vi "CheesyDrive.vi"(6 "Quickturn":bool, 7 "SlowMode":u32, 8 "Fast Mode":bool, 10 "Wheel":dbl(slide)=-0.015748031496062992 scale=-1.0..1.0, 11 "Throttle":dbl(slide)=0.007874015748031496 scale=-1.0..1.0) -> (2 "Right PWM":dbl, 3 "Left PWM":dbl)   [LabVIEW 2018]
doc: "Implements CheesyDrive. CheesyDrive means that the turn joystick controls the radius of turning instead of the rate of turning. Also implements QuickStop and QuickTurn."
uses:
  Robot-Project/Arm/Implementation/Arm Published Globals.vi
panel:
  in  "ArrayOfSlownesss":T1(array[cluster])=[{"MaxSpeedSlow"=1.0, "SlowRate"=5.0, "MaxTurnSlow"=1.0, "MaxTurnRateSlow"=8.0}, {"MaxSpeedSlow"=0.6, "SlowRate"=4.0, "MaxTurnSlow"=0.8, "MaxTurnRateSlow"=10.0}, {"MaxSpeedSlow"=0.4, "SlowRate"=3.0, "MaxTurnSlow"=0.75, "MaxTurnRateSlow"=10.0}]
  in  "PointsTurn":cluster{"X":dbl, "Y":dbl}[](array[cluster])=[{"X"=0.0, "Y"=0.0}, {"X"=0.04, "Y"=0.0}, {"X"=0.041, "Y"=0.01}, {"X"=0.6, "Y"=0.3}, {"X"=1.0, "Y"=1.0}]
  in  "PointsQuickTurn":cluster{"X":dbl, "Y":dbl}[](array[cluster])=[{"X"=0.0, "Y"=0.0}, {"X"=0.05, "Y"=0.05}, {"X"=1.0, "Y"=0.6}]
  in  "PointsThrottle":cluster{"X":dbl, "Y":dbl}[](array[cluster])=[{"X"=0.0, "Y"=0.0}, {"X"=0.025, "Y"=0.0}, {"X"=1.0, "Y"=0.75}]
  in  "QSMult":dbl=0.12
  in  "WheelNonLinearity":dbl=0.01
  in  "negInertiaScalar":dbl=4.0
  in  "alpha":dbl=0.1
  out "QuickStop Value":dbl(graph)
  in  "Sensitivty":dbl=1.0
  # "These are the inputs and outputs\nNot configuration"
  # "Check block diagram for details on these"
  # "normal"
  # "Switch"
  # "Scale"
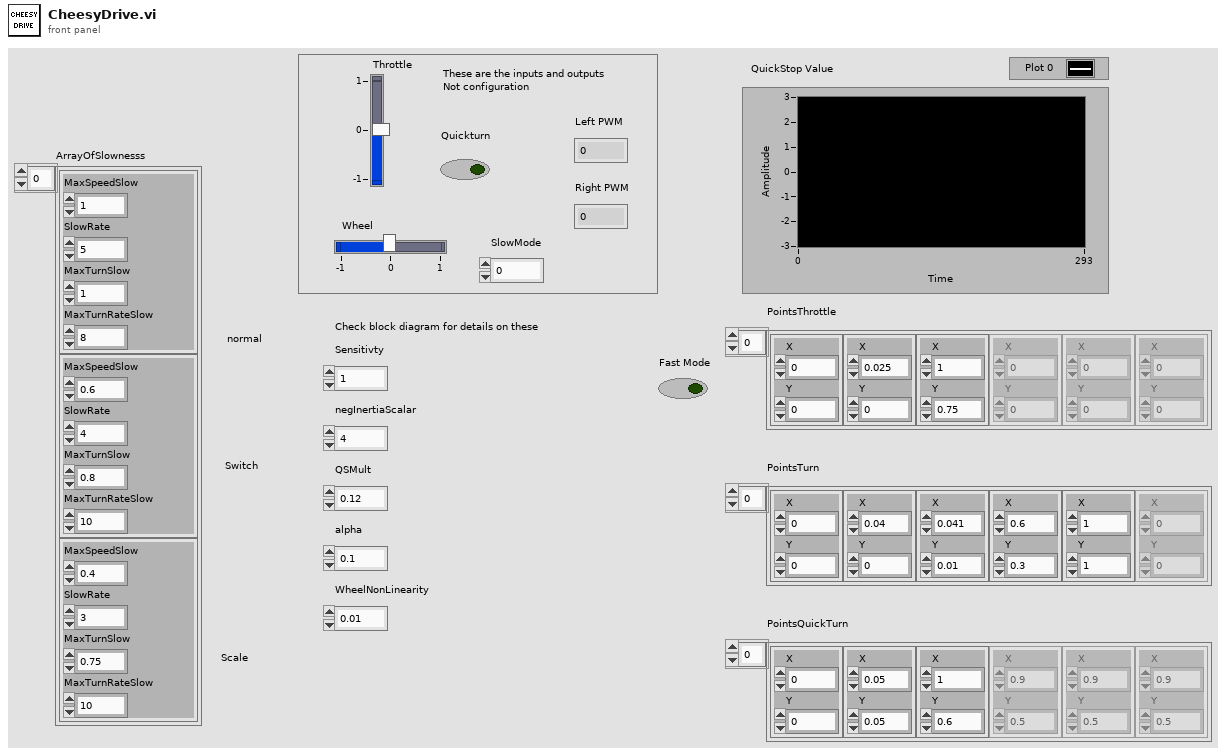
[diagram p1: front panel]
types:
  T1 = cluster{"MaxSpeedSlow":dbl, "SlowRate":dbl, "MaxTurnSlow":dbl, "MaxTurnRateSlow":dbl}[]
  T2 = cluster{"MaxSpeedSlow":dbl, "SlowRate":dbl, "MaxTurnSlow":dbl, "MaxTurnRateSlow":dbl}
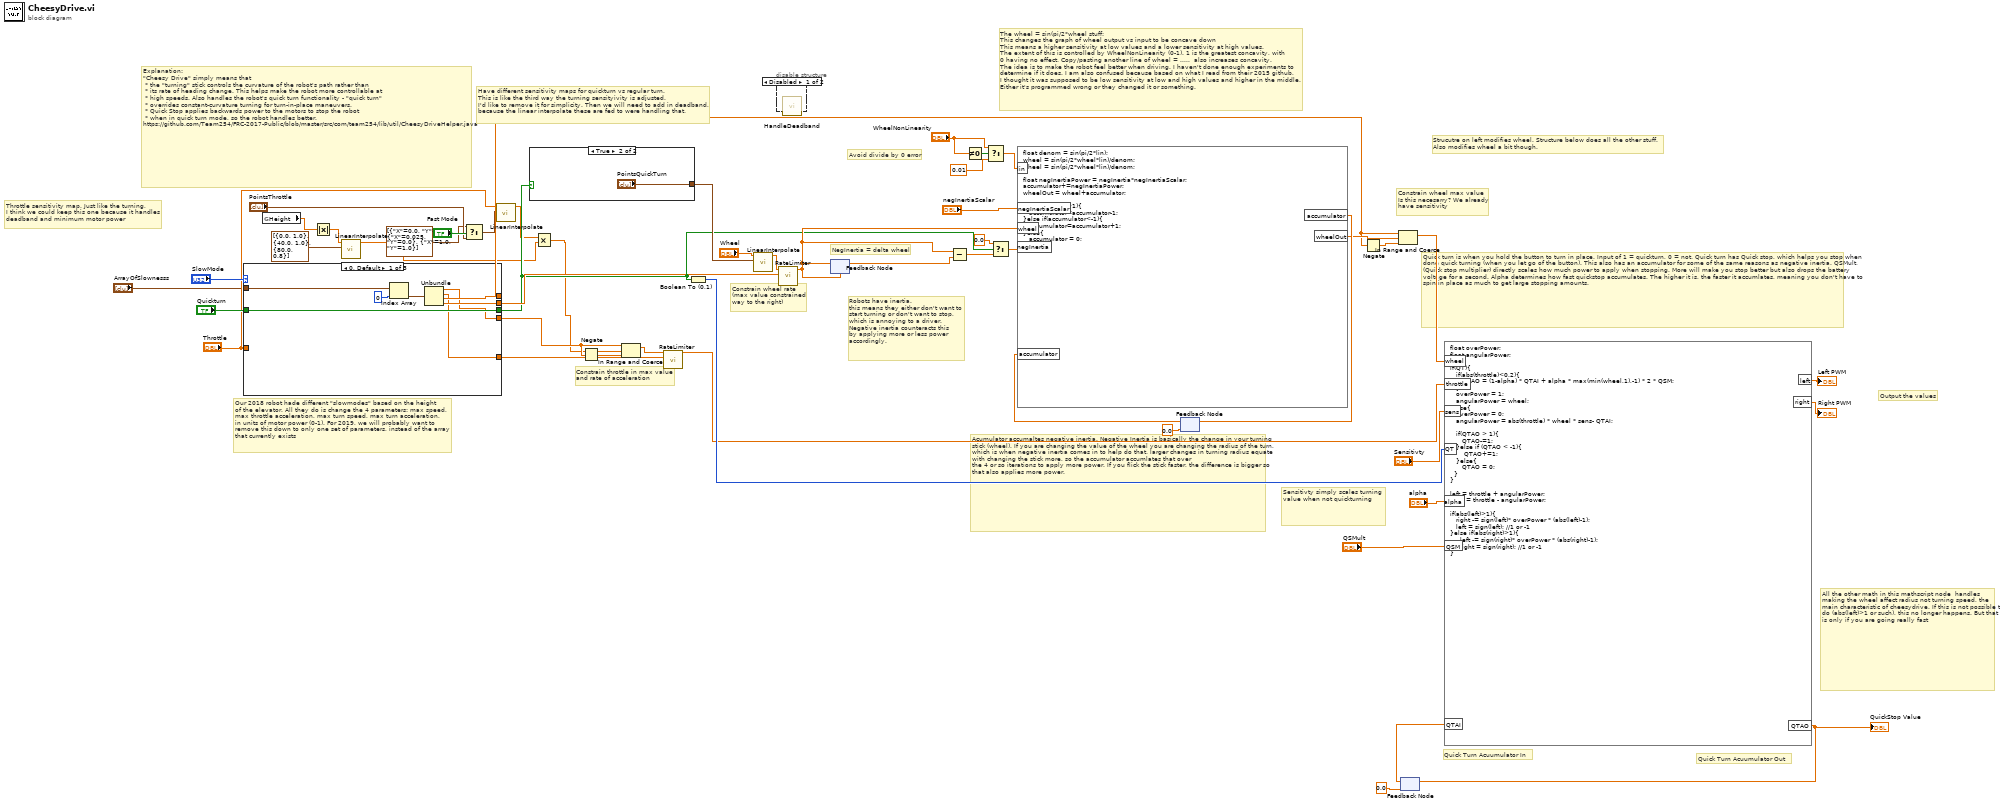
[diagram p0: block diagram]
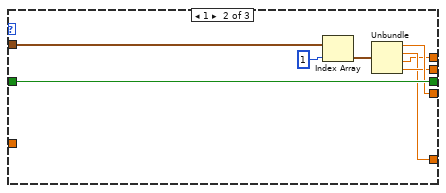
[diagram p3: hidden frame]
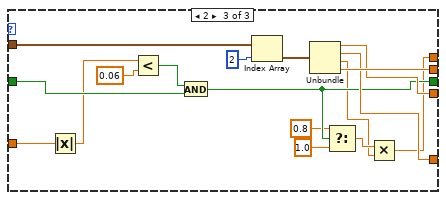
[diagram p4: hidden frame]
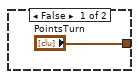
[diagram p5: hidden frame]
diagram:
  # "Strucutre on left modifies wheel. Structure below does all the other stuff.\nAlso modifies wheel a bit though."
  # "Sensitivty simply scales turning value when not quickturning"
  # "All the other math in this mathscript node  handles making the wheel affect radius not turning speed, the main characteristic of cheesydrive. If this is not possible to do (abs(left)>1 or such), this no longer happens. But that is only if you are going really fast"
  # "Quick turn is when you hold the button to turn in place. Input of 1 = quickturn, 0 = not. Quick turn has Quick stop, which helps you stop when done quick turning (when you let go of the button). This also has an accumulator for some of the same reasons as negative inertia. QSMult, (Quick stop multiplier) directly scales how much power to apply when stopping. More will make you stop better but also drops the battery voltage for a second. Alpha determines how fast quickstop accumulates. The higher it is, the faster it accumlates, meaning you don't have to spin in place as much to get large stopping amounts."
  # "Output the values"
  # "Acumulator accumaltes negative inertia. Negative Inertia is basically the change in your turning stick (wheel). If you are changing the value of the wheel you are changing the radius of the turn, which is when negative inertia comes in to help do that. larger changes in turning radius equate with changing the stick more, so the accumulator accumlates that over\nthe 4 or so iterations to apply more power. If you flick the stick faster, the difference is bigger so that also applies more power."
  # "The wheel = sin(pi/2*wheel stuff:\nThis changes the graph of wheel output vs input to be concave down\nThis means a higher sensitivity at low values and a lower sensitivity at high values.\nThe extent of this is controlled by WheelNonLinearity (0-1). 1 is the greatest concavity, with\n0 having no effect. Copy/pasting another line of wheel = .....  also increases concavity.\nThe idea is to make the robot feel better when driving. I haven't done enough experiments to \ndetermine if it does. I am also confused because based on what I read from their 2015 github,\nI thought it was supposed to be low sensitivity at low and high values and higher in the middle.\nEither it's programmed wrong or they changed it or something."
  # "Constrain wheel max value\nIs this necesarry? We already\nhave sensitivity"
  # "Constrain wheel rate\n(max value constrained\nway to the right)"
  # "Throttle sensitivity map. Just like the turning,\nI think we could keep this one because it handles\ndeadband and minimum motor power"
  # "Have different sensitivity maps for quickturn vs regular turn.\nThis is like the third way the turning sensityivity is adjusted. \nI'd like to remove it for simplicity. Then we will need to add in deadband,\nbecause the linear interpolate these are fed to were handling that."
  # "Robots have inertia.\nthis means they either don't want to\nstart turning or don't want to stop,\nwhich is annoying to a driver. \nNegative inertia counteracts this\nby applying more or less power\naccordingly."
  # "Constrain throttle in max value\nand rate of acceleration"
  # "Our 2018 robot hade different \"slowmodes\" based on the height\nof the elevator. All they do is change the 4 parameters: max speed,\nmax throttle acceleration, max turn speed, max turn acceleration,\nin units of motor power (0-1). For 2019, we will probably want to\nremove this down to only one set of parameters, instead of the array\nthat currently exists"
  # "Avoid divide by 0 error"
  # "NegInertia = delta wheel"
  # "Explanation:\n\"Cheesy Drive\" simply means that\n * the \"turning\" stick controls the curvature of the robot's path rather than\n * its rate of heading change. This helps make the robot more controllable at\n * high speeds. Also handles the robot's quick turn functionality - \"quick turn\"\n * overrides constant-curvature turning for turn-in-place maneuvers.\n * Quick Stop applies backwards power to the motors to stop the robot\n * when in quick turn mode, so the robot handles better.\nhttps://github.com/Team254/FRC-2017-Public/blob/master/src/com/team254/lib/util/CheesyDriveHelper.java"
  # "Quick Turn Acuumulator Out"
  # "Quick Turn Acuumulator In"
  n1 = case shown="0, Default" "SlowMode" {
    tunnel: [w51 w60 w74] -> w30
    tunnel: [w52 w62 w76] -> w15
    tunnel: [w53 w59 w67] -> w28
    tunnel: [w54 w61 w77] -> w26
    tunnel: "Quickturn" -> [w58 w66 w83]
    tunnel: [w58 w66 w71] -> w19
    tunnel: "Throttle" -> [_ _ w75]
    tunnel: "ArrayOfSlownesss" -> [w55 w63 w80]
    frame 0, Default {
      n2 = Index Array(array=w55, index=0) -> (element=w56:T2)
      n3 = Unbundle(w56) -> ("MaxSpeedSlow"=w52:dbl, "SlowRate"=w51:dbl, "MaxTurnSlow"=w53:dbl, "MaxTurnRateSlow"=w54:dbl)
    }
    frame 1 {
      n4 = Index Array(array=w63, index=1) -> (element=w64:T2)
      n5 = Unbundle(w64) -> ("MaxSpeedSlow"=w62:dbl, "SlowRate"=w60:dbl, "MaxTurnSlow"=w59:dbl, "MaxTurnRateSlow"=w61:dbl)
    }
    frame 2 {
      n6 = Absolute Value(x=w75) -> (abs(x)=w73:dbl)
      n7 = Less?(x=w73, y=0.06) -> (x < y?=w82:bool)
      n8 = And(x=w82, y=w83) -> (x .and. y?=w71:bool)
      n9 = Index Array(array=w80, index=2) -> (element=w78:T2)
      n10 = Unbundle(w78) -> ("MaxSpeedSlow"=w76:dbl, "SlowRate"=w74:dbl, "MaxTurnSlow"=w68:dbl, "MaxTurnRateSlow"=w77:dbl)
      n11 = Select(t=0.8, s=w71, f=1.0) -> (s? t:f=w69:dbl)
      n12 = Multiply(x=w69, y=w68) -> (x*y=w67:dbl)
    }
  }
  n13 = global read "Arm Published Globals.vi" "Height"() -> (w3:dbl)
  n14 = Absolute Value(x=w3) -> (abs(x)=w2:dbl)
  n15 = call "LinearInterpolate.vi"("Points"=cluster{"X":dbl, "Y":dbl}[] [{"X"=0.0, "Y"=1.0}, {"X"=40.0, "Y"=1.0}, {"X"=80.0, "Y"=0.8}], "Value"=w2) -> ("Output"=w1:dbl)  [unwired: 9 in]
  n16 = Select(t=cluster{"X":dbl, "Y":dbl}[] [{"X"=0.0, "Y"=0.0}, {"X"=0.025, "Y"=0.0}, {"X"=1.0, "Y"=1.0}] ("PointsThrottle"), s="Fast Mode", f="PointsThrottle") -> (s? t:f=w7:cluster{"X":dbl, "Y":dbl}[])
  n17 = call "LinearInterpolate.vi"("Points"=w7, "Value"="Throttle") -> ("Output"=w5:dbl)  [unwired: 9 in]
  n18 = case shown="True" w19 {
    tunnel: ["PointsTurn" "PointsQuickTurn"] -> w32
    frame False {
    }
    frame True {
    }
  }
  n19 = Multiply(x=w5, y=w1) -> (x*y=w4:dbl)
  n20 = Negate(x=w15) -> (-x=w16:dbl)
  n21 = In Range and Coerce(upper limit=w15, x=w4, lower limit=w16) -> (coerced(x)=w17:dbl)  [unwired: 1 out]
  n22 = call "RateLimiter.vi"("Max dx/dt"=w30, "Input"=w17) -> ("Output"=w44:dbl)  [unwired: 9 in]
  n23 = Boolean To (0,1)(Boolean=w19) -> (0, 1=w48:i16)
  n24 = call "LinearInterpolate.vi"("Points"=w32, "Value"="Wheel") -> ("Output"=w27:dbl)  [unwired: 9 in]
  n25 = disable-structure shown="Disabled" {
    frame Disabled {
      n26 = call "HandleDeadband.vi"() -> ()  [unwired: 11 in, 1 out]
    }
    frame Enabled {
    }
  }
  n27 = call "RateLimiter.vi"("Max dx/dt"=w26, "Input"=w27) -> ("Output"=w33:dbl)  [unwired: 9 in]
  n28 = feedback #1(w33) -> (w41:dbl)
  n29 = feedback-in #1(w33) -> ()
  n30 = Subtract(x=w33, y=w41) -> (x-y=w24:dbl)
  n31 = Not Equal To 0?(x="WheelNonLinearity") -> (x != 0?=w14:bool)
  n32 = Select(t="WheelNonLinearity", s=w14, f=0.01) -> (s? t:f=w11:dbl)
  n33 = Select(t=0.0, s=w19, f=w24) -> (s? t:f=w25:dbl)
  n34 = feedback #2(0.0 ("Wheel")) -> (w40:dbl)
  n35 = formula code="float denom = sin(pi/2*lin);\nwheel = sin(pi/2*wheel*lin)/denom;\nwheel = sin(pi/2*wheel*lin)/denom;\n\nfloat negInertiaPower = negInertia*negInertiaScalar;\naccumulator+=negInertiaPower;\nwheelOut = wheel+accumulator;\n\nif(accumulator>1){\n   accumulator=accumulator-1;\n}else if(accumulator<-1){\n   accumulator=accumulator+1;\n}else{\n   accumulator = 0;\n}"("wheel"=w33, "negInertia"=w25, "accumulator"=w40, "negInertiaScalar"="negInertiaScalar", "lin"=w11) -> ("accumulator"=w38:dbl, "wheelOut"=w35:dbl)
  n36 = feedback-in #2(w38) -> ()
  n37 = Negate(x=w28) -> (-x=w29:dbl)
  n38 = In Range and Coerce(upper limit=w28, x=w35, lower limit=w29) -> (coerced(x)=w36:dbl)  [unwired: 1 out]
  n39 = feedback #3(0.0 ("QTAccumulatorO")) -> (w46:dbl)
  n40 = formula code="float overPower;\nfloat angularPower;\n\nif(QT){\n   if(abs(throttle)<0.2){\n      QTAO = (1-alpha) * QTAI + alpha * max(min(wheel,1),-1) * 2 * QSM;\n   }\n   overPower = 1;\n   angularPower = wheel;\n}else{\n   overPower = 0;\n   angularPower = abs(throttle) * wheel * sens- QTAI;\n\n   if(QTAO > 1){\n      QTAO-=1;\n   }else if (QTAO < -1){\n       QTAO+=1;\n   }else{\n      QTAO = 0;\n  }\n}\n\nleft = throttle + angularPower;\nright = throttle - angularPower;\n\nif(abs(left)>1){\n   right -= sign(left)* overPower * (abs(left)-1);\n   left = sign(left); //1 or -1\n}else if(abs(right)>1){\n     left -= sign(right)* overPower * (abs(right)-1);\n     right = sign(right); //1 or -1 \n}"("wheel"=w36, "throttle"=w44, "sens"="Sensitivty", "QT"=w48, "alpha"="alpha", "QTAI"=w46, "QSM"="QSMult") -> ("left"=→"Left PWM":dbl, "right"=→"Right PWM":dbl, "QTAO"=w49:dbl)
  "QuickStop Value" <- w49
  n41 = feedback-in #3(w49) -> ()
